vi "draw the stage.vi"(6 "stepper motor state":T1, 7 "slider setter action":T2, 8 "set":refnum<vi>, 9 "angle":refnum<vi>, 10 "current pos...":refnum<vi>, 11 "XY Graph":refnum<vi>) -> ()   [LabVIEW 2018]
uses:
  slider setter action.ctl
  stepper motor state.ctl
  2Dwindow.ctl
  slider action.ctl
  cursor action.ctl
  generate linear region.vi
panel:
  out "angle 2":dbl(slide)=743.9484386624194 scale=-90.0..90.0 scale format="%^#6_6g"
  out "current pos...  2":dbl(slide) scale=0.0..16000.0
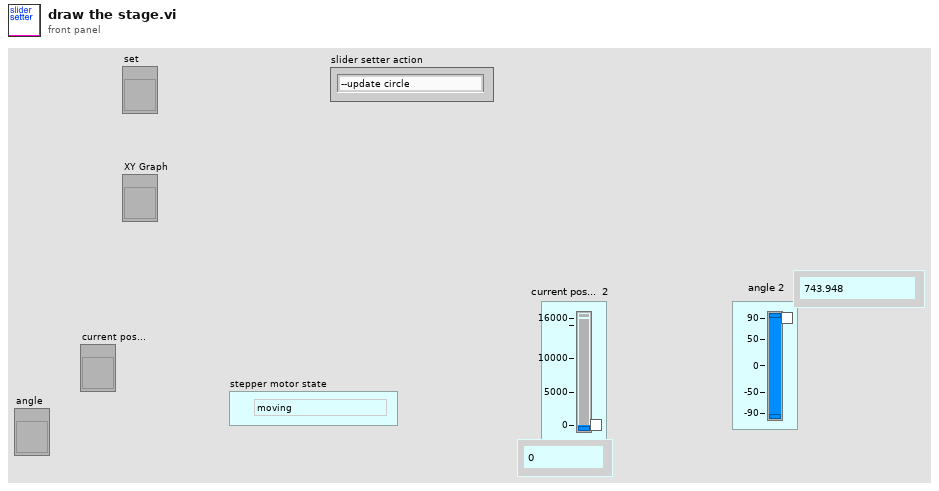
[diagram p1: front panel]
types:
  T1 = typedef "stepper motor state.ctl" = enum16{"moving", "stopped"}
  T2 = typedef "slider setter action.ctl" = enum16{"--update circle", "set slider moves", "cursor moves", "current pos changed", "init"}
  T3 = typedef "2Dwindow.ctl" = cluster{"window y":dbl, "center x":dbl, "center y":dbl, "window x":dbl}
  T4 = typedef "slider action.ctl" = enum16{"check", "copy range", "set", "set ratio"}
  T5 = typedef "cursor action.ctl" = enum16{"range", "read", "write", "check", "zoom out", "smart zoom out", "zoom to aspect ratio 1", "zoom to win", "zoom out 20%", "zoom in 20%", "-empty", "smart zoom out&aspect", "move range left 20%", "move range right 20%", "move range up 20%", "move range down 20%", "zoom to X win", "zoom to Y win", "zoom out X", "zoom out Y", "zoom in X", "zoom in Y", "check plot scale"}
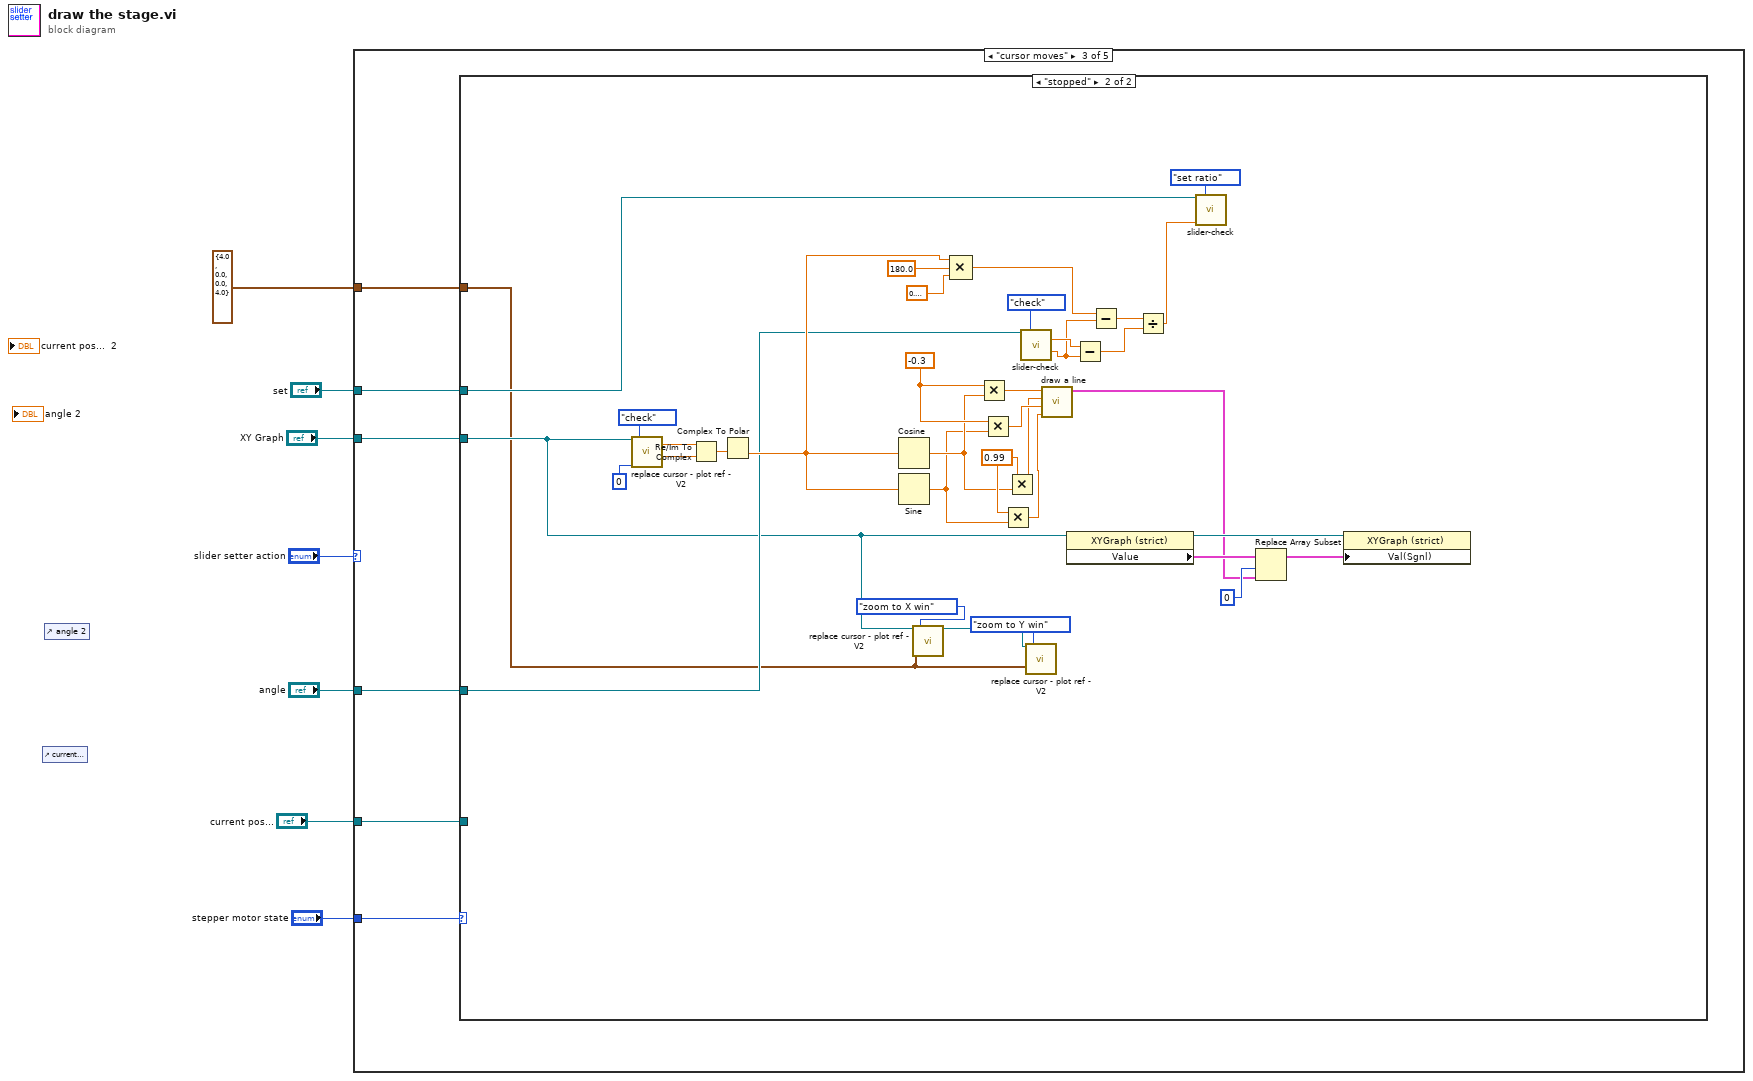
[diagram p0: block diagram]
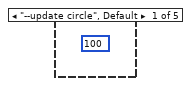
[diagram p2: hidden frame]
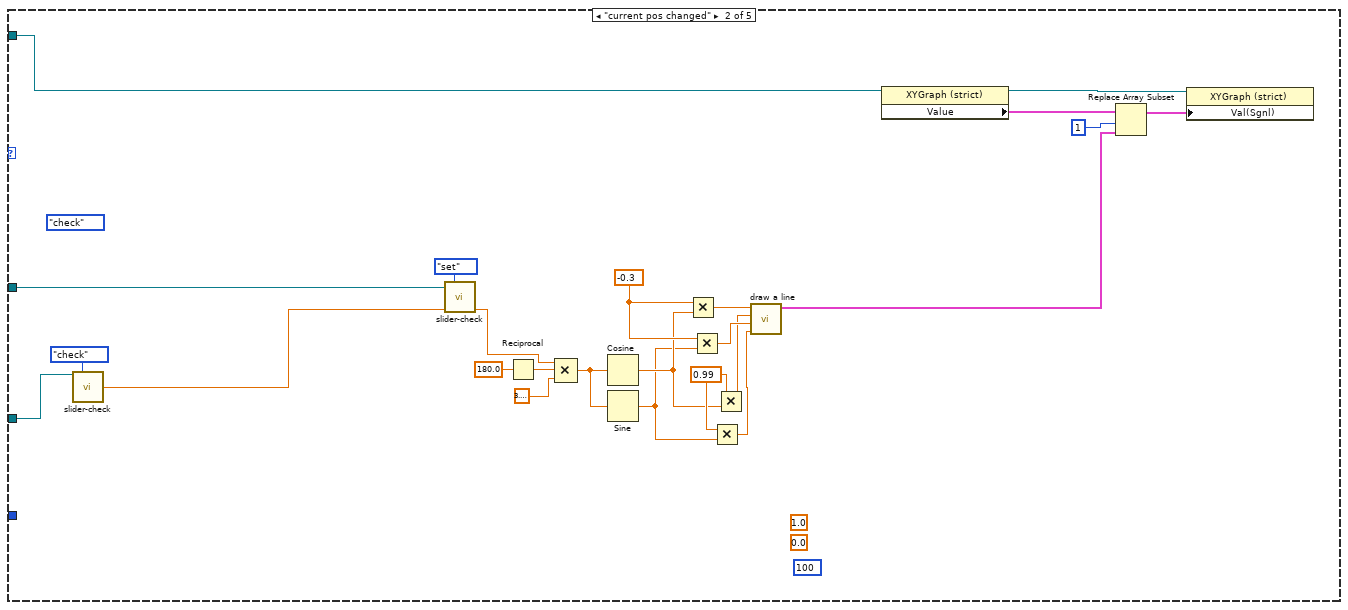
[diagram p3: hidden frame]
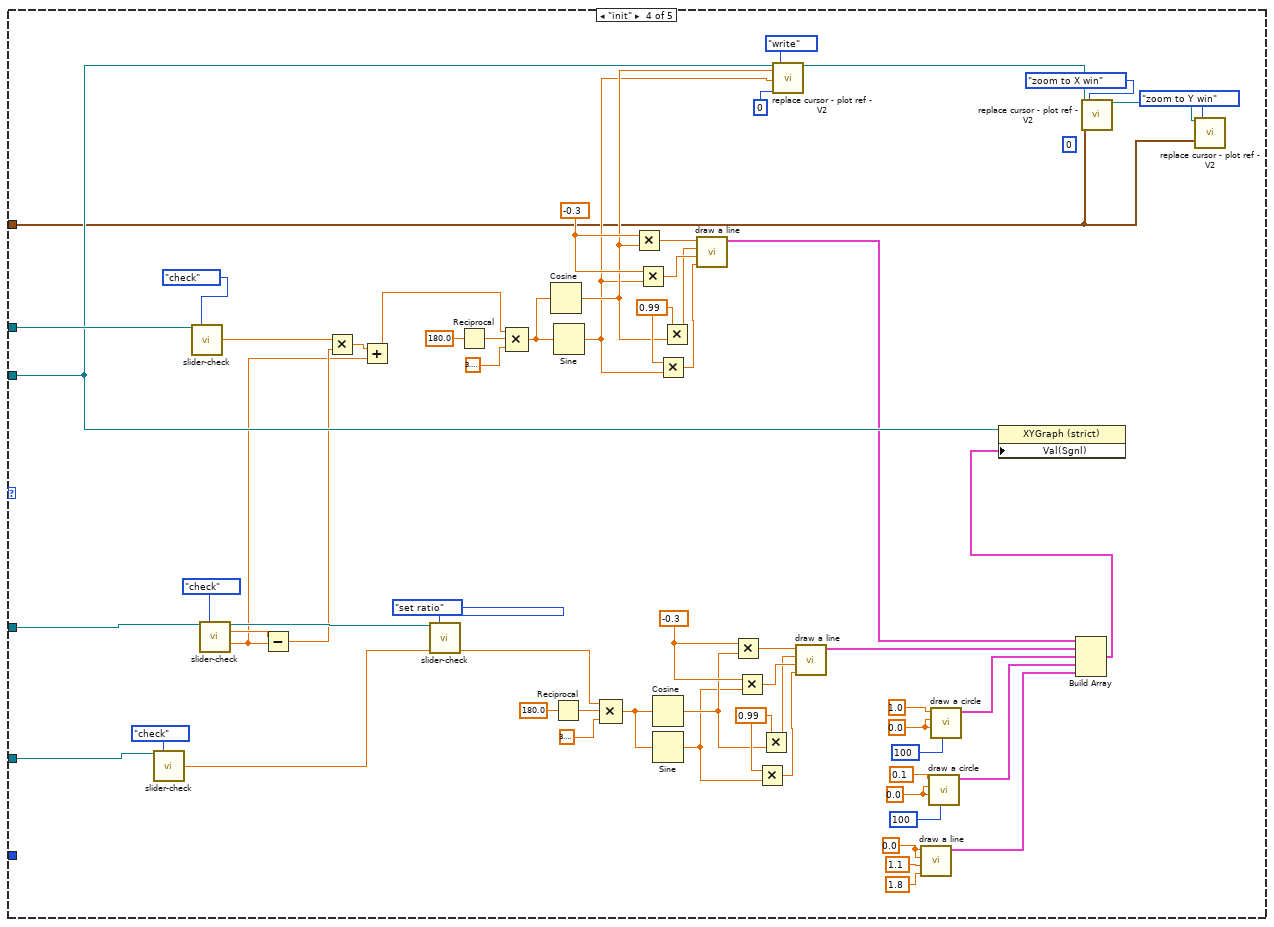
[diagram p5: hidden frame]
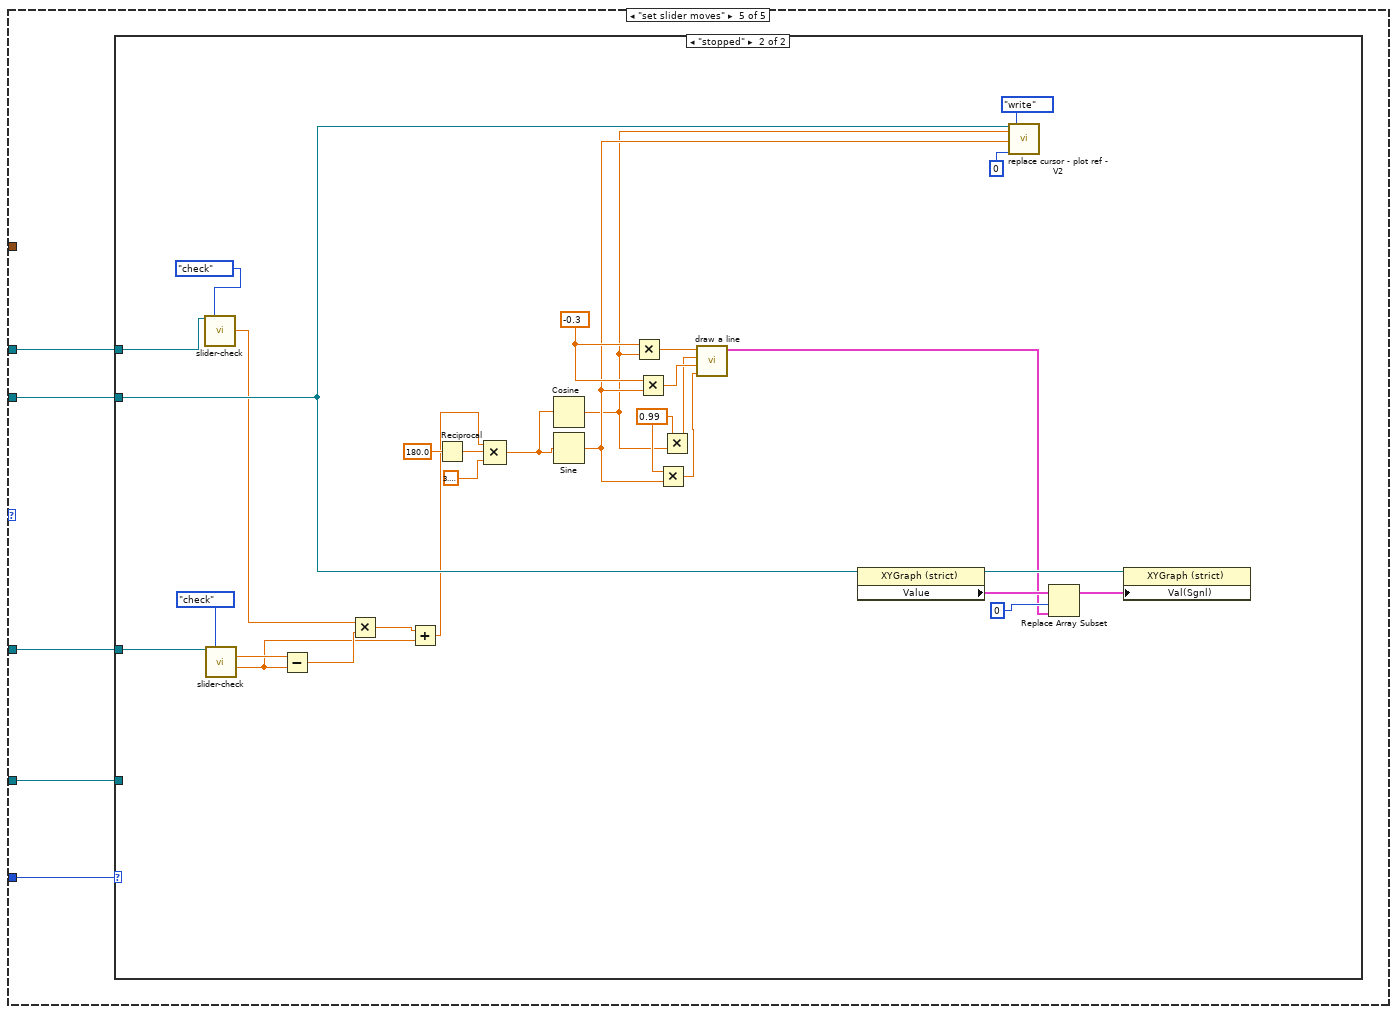
[diagram p6: hidden frame]
diagram:
  n1 = control-ref of="current pos...  2"() -> ()  [unwired: 1 out]
  n2 = control-ref of="angle 2"() -> ()  [unwired: 1 out]
  n3 = case shown="\"cursor moves\"" "slider setter action" {
    tunnel: "angle" -> [_ w9 w36 w136 w140]
    tunnel: "current pos..." -> [_ w18 w35 w135 w139]
    tunnel: "XY Graph" -> [_ w16 w37 w93 w141]
    tunnel: "set" -> [_ _ w34 w134 w138]
    tunnel: "stepper motor state" -> [_ _ w33 _ w137]
    tunnel: T3 {"window y"=4.0, "center x"=0.0, "center y"=0.0, "window x"=4.0} ("window IN") -> [_ _ w32 w74 _]
    frame "--update circle", Default {
      (unwired) 100 ("number of points")
    }
    frame "current pos changed" {
      (unwired) slider_action."check" ("slider action")
      w24 = 0.99 ("x")
      w26 = -0.3 ("x")
      (unwired) 100 ("number of points")
      (unwired) 1.0 ("radius")
      (unwired) 0.0 ("center x")
      n4 = call "slider-check.vi"("slider"=w18, "slider action"=slider_action."check") -> ("rel OUT"=w11:dbl)  [unwired: 9 in, 4 out]
      n5 = call "slider-check.vi"("slider"=w9, "slider action"=slider_action."set", "value IN"=w11) -> ("value OUT"=w10:dbl)  [unwired: 8 in, 4 out]
      n6 = Reciprocal(x=180.0 ("x0")) -> (1/x=w30:dbl)
      n7 = Compound Arithmetic op=MULTIPLY(w10, w30, 3.141592653589793) -> (w28:dbl)
      n8 = Cosine(x=w28) -> (cos(x)=w21:dbl)
      n9 = Sine(x=w28) -> (sin(x)=w20:dbl)
      n10 = Multiply(x=w26, y=w21) -> (x*y=w27:dbl)
      n11 = Multiply(x=w26, y=w20) -> (x*y=w25:dbl)
      n12 = Multiply(x=w24, y=w20) -> (x*y=w22:dbl)
      n13 = Multiply(x=w24, y=w21) -> (x*y=w23:dbl)
      n14 = call "draw a line.vi"("y1"=w22, "y0"=w25, "x1"=w23, "x0"=w27) -> ("output cluster"=w8:cluster{dbl[], dbl[]})  [unwired: 7 in]
      n15 = property class="XYGraph (strict)"(reference=w16) -> (reference out=w15:refnum<vi>, "Value"=w14:cluster{dbl[], dbl[]}[])  [unwired: 1 in, 1 out]
      n16 = Replace Array Subset(array=w14, new element=w8, index=1) -> (w13:cluster{dbl[], dbl[]}[])
      n17 = property class="XYGraph (strict)"(reference=w15, "Val(Sgnl)"=w13) -> ()  [unwired: 1 in, 2 out]
    }
    frame "cursor moves" {
      n18 = case shown="\"stopped\"" w33 {
        tunnel: w37 -> [_ w42]
        tunnel: w36 -> [_ w50]
        tunnel: w35 -> [_ _]
        tunnel: w34 -> [_ w49]
        tunnel: w32 -> [_ w38]
        frame "moving", Default {
        }
        frame "stopped" {
          w70 = 0.99 ("x")
          w72 = -0.3 ("x")
          n19 = call "replace cursor - plot ref - V2.vi"("Plot ref in"=w42, "cursor index"=0, "cursor action"=cursor_action."check") -> ("read X"=w63:dbl, "read Y"=w62:dbl)  [unwired: 13 in, 2 out]
          n20 = Re/Im To Complex(1:w62, 2:w63) -> (0:w61:cdb)
          n21 = Complex To Polar(r * e^(i*theta)=w61) -> (theta=w54:dbl)  [unwired: 1 out]
          n22 = Cosine(x=w54) -> (cos(x)=w67:dbl)
          n23 = Sine(x=w54) -> (sin(x)=w66:dbl)
          n24 = call "replace cursor - plot ref - V2.vi"("Plot ref in"=w42, "window IN"=w38, "cursor action"=cursor_action."zoom to X win") -> ("Plot ref out"=w40:refnum<vi>)  [unwired: 13 in, 3 out]
          n25 = Compound Arithmetic op=MULTIPLY(w54, 180.0 ("x0"), 0.3183098861837907) -> (w46:dbl)
          n26 = Multiply(x=w72, y=w67) -> (x*y=w73:dbl)
          n27 = Multiply(x=w72, y=w66) -> (x*y=w71:dbl)
          n28 = Multiply(x=w70, y=w66) -> (x*y=w68:dbl)
          n29 = Multiply(x=w70, y=w67) -> (x*y=w69:dbl)
          n30 = call "slider-check.vi"("slider"=w50, "slider action"=slider_action."check") -> ("max"=w48:dbl, "min"=w47:dbl)  [unwired: 9 in, 3 out]
          n31 = call "replace cursor - plot ref - V2.vi"("Plot ref in"=w40, "window IN"=w38, "cursor action"=cursor_action."zoom to Y win") -> ()  [unwired: 13 in, 4 out]
          n32 = call "draw a line.vi"("y1"=w68, "y0"=w71, "x1"=w69, "x0"=w73) -> ("output cluster"=w56:cluster{dbl[], dbl[]})  [unwired: 7 in]
          n33 = property class="XYGraph (strict)"(reference=w42) -> (reference out=w60:refnum<vi>, "Value"=w59:cluster{dbl[], dbl[]}[])  [unwired: 1 in, 1 out]
          n34 = Subtract(x=w48, y=w47) -> (x-y=w44:dbl)
          n35 = Subtract(x=w46, y=w47) -> (x-y=w45:dbl)
          n36 = Divide(x=w45, y=w44) -> (x/y=w43:dbl)
          n37 = call "slider-check.vi"("slider"=w49, "slider action"=slider_action."set ratio", "value IN"=w43) -> ()  [unwired: 8 in, 5 out]
          n38 = Replace Array Subset(array=w59, new element=w56, index=0) -> (w58:cluster{dbl[], dbl[]}[])
          n39 = property class="XYGraph (strict)"(reference=w60, "Val(Sgnl)"=w58) -> ()  [unwired: 1 in, 2 out]
        }
      }
    }
    frame "init" {
      (unwired) 0 ("cursor index")
      w103 = 0.99 ("x")
      w105 = -0.3 ("x")
      w115 = 0.0 ("center x")
      w120 = 0.99 ("x")
      w122 = -0.3 ("x")
      w130 = 0.0 ("x0")
      w133 = 0.0 ("center x")
      n40 = call "slider-check.vi"("slider"=w135, "slider action"=slider_action."check") -> ("rel OUT"=w95:dbl)  [unwired: 9 in, 4 out]
      n41 = call "slider-check.vi"("slider"=w134, "slider action"=slider_action."check") -> ("rel OUT"=w90:dbl)  [unwired: 9 in, 4 out]
      n42 = call "slider-check.vi"("slider"=w136, "slider action"=slider_action."check") -> ("slider OUT"=w108:refnum<vi>, "max"=w89:dbl, "min"=w86:dbl)  [unwired: 9 in, 2 out]
      n43 = Subtract(x=w89, y=w86) -> (x-y=w88:dbl)
      n44 = Multiply(x=w90, y=w88) -> (x*y=w87:dbl)
      n45 = Add(x=w87, y=w86) -> (x+y=w82:dbl)
      n46 = call "slider-check.vi"("slider"=w108, "slider action"=slider_action."set ratio", "value IN"=w95) -> ("value OUT"=w94:dbl)  [unwired: 8 in, 4 out]
      n47 = Reciprocal(x=180.0 ("x0")) -> (1/x=w84:dbl)
      n48 = Compound Arithmetic op=MULTIPLY(w82, w84, 3.141592653589793) -> (w81:dbl)
      n49 = Cosine(x=w81) -> (cos(x)=w80:dbl)
      n50 = Reciprocal(x=180.0 ("x0")) -> (1/x=w126:dbl)
      n51 = Sine(x=w81) -> (sin(x)=w79:dbl)
      n52 = Compound Arithmetic op=MULTIPLY(w94, w126, 3.141592653589793) -> (w124:dbl)
      n53 = Multiply(x=w105, y=w80) -> (x*y=w106:dbl)
      n54 = Multiply(x=w105, y=w79) -> (x*y=w104:dbl)
      n55 = Cosine(x=w124) -> (cos(x)=w112:dbl)
      n56 = Sine(x=w124) -> (sin(x)=w111:dbl)
      n57 = Multiply(x=w103, y=w79) -> (x*y=w101:dbl)
      n58 = Multiply(x=w103, y=w80) -> (x*y=w102:dbl)
      n59 = call "draw a line.vi"("y1"=w101, "y0"=w104, "x1"=w102, "x0"=w106) -> ("output cluster"=w92:cluster{dbl[], dbl[]})  [unwired: 7 in]
      n60 = Multiply(x=w122, y=w112) -> (x*y=w123:dbl)
      n61 = Multiply(x=w122, y=w111) -> (x*y=w121:dbl)
      n62 = Multiply(x=w120, y=w111) -> (x*y=w118:dbl)
      n63 = Multiply(x=w120, y=w112) -> (x*y=w119:dbl)
      n64 = call "replace cursor - plot ref - V2.vi"("Plot ref in"=w93, "new X"=w80, "new  Y"=w79, "cursor index"=0, "cursor action"=cursor_action."write") -> ("Plot ref out"=w75:refnum<vi>)  [unwired: 11 in, 3 out]
      n65 = call "draw a line.vi"("y1"=w118, "y0"=w121, "x1"=w119, "x0"=w123) -> ("output cluster"=w96:cluster{dbl[], dbl[]})  [unwired: 7 in]
      n66 = call "draw a line.vi"("y1"=1.8 ("x0"), "y0"=1.1 ("x0"), "x1"=w130, "x0"=w130) -> ("output cluster"=w116:cluster{dbl[], dbl[]})  [unwired: 7 in]
      n67 = call "draw a circle.vi"("number of points"=100, "center Y"=w115, "center x"=w115, "radius"=0.1) -> ("output cluster"=w97:cluster{dbl[], dbl[]})  [unwired: 7 in]
      n68 = call "draw a circle.vi"("number of points"=100, "center Y"=w133, "center x"=w133, "radius"=1.0) -> ("output cluster"=w117:cluster{dbl[], dbl[]})  [unwired: 7 in]
      n69 = Build Array(w92, w96, w117, w97, w116) -> (w91:cluster{dbl[], dbl[]}[])
      n70 = property class="XYGraph (strict)"(reference=w93, "Val(Sgnl)"=w91) -> ()  [unwired: 1 in, 2 out]
      n71 = call "replace cursor - plot ref - V2.vi"("Plot ref in"=w75, "window IN"=w74, "cursor action"=cursor_action."zoom to X win") -> ("Plot ref out"=w77:refnum<vi>)  [unwired: 13 in, 3 out]
      n72 = call "replace cursor - plot ref - V2.vi"("Plot ref in"=w77, "window IN"=w74, "cursor action"=cursor_action."zoom to Y win") -> ()  [unwired: 13 in, 4 out]
    }
    frame "set slider moves" {
      n73 = case shown="\"stopped\"" w137 {
        tunnel: w141 -> [_ w163]
        tunnel: w140 -> [_ w156]
        tunnel: w139 -> [_ _]
        tunnel: w138 -> [_ w154]
        frame "moving", Default {
        }
        frame "stopped" {
          w168 = 0.99 ("x")
          w170 = -0.3 ("x")
          n74 = call "slider-check.vi"("slider"=w154, "slider action"=slider_action."check") -> ("rel OUT"=w151:dbl)  [unwired: 9 in, 4 out]
          n75 = call "slider-check.vi"("slider"=w156, "slider action"=slider_action."check") -> ("max"=w153:dbl, "min"=w149:dbl)  [unwired: 9 in, 3 out]
          n76 = Subtract(x=w153, y=w149) -> (x-y=w152:dbl)
          n77 = Multiply(x=w151, y=w152) -> (x*y=w150:dbl)
          n78 = Add(x=w150, y=w149) -> (x+y=w145:dbl)
          n79 = Reciprocal(x=180.0 ("x0")) -> (1/x=w147:dbl)
          n80 = Compound Arithmetic op=MULTIPLY(w145, w147, 3.141592653589793) -> (w144:dbl)
          n81 = Cosine(x=w144) -> (cos(x)=w142:dbl)
          n82 = Sine(x=w144) -> (sin(x)=w143:dbl)
          n83 = Multiply(x=w170, y=w142) -> (x*y=w171:dbl)
          n84 = Multiply(x=w170, y=w143) -> (x*y=w169:dbl)
          n85 = Multiply(x=w168, y=w143) -> (x*y=w166:dbl)
          n86 = Multiply(x=w168, y=w142) -> (x*y=w167:dbl)
          n87 = call "draw a line.vi"("y1"=w166, "y0"=w169, "x1"=w167, "x0"=w171) -> ("output cluster"=w158:cluster{dbl[], dbl[]})  [unwired: 7 in]
          n88 = property class="XYGraph (strict)"(reference=w163) -> (reference out=w160:refnum<vi>, "Value"=w162:cluster{dbl[], dbl[]}[])  [unwired: 1 in, 1 out]
          n89 = call "replace cursor - plot ref - V2.vi"("Plot ref in"=w163, "new X"=w142, "new  Y"=w143, "cursor index"=0, "cursor action"=cursor_action."write") -> ()  [unwired: 11 in, 4 out]
          n90 = Replace Array Subset(array=w162, new element=w158, index=0) -> (w161:cluster{dbl[], dbl[]}[])
          n91 = property class="XYGraph (strict)"(reference=w160, "Val(Sgnl)"=w161) -> ()  [unwired: 1 in, 2 out]
        }
      }
    }
  }
